vi "CheckState.vi"(8 "Error In":errorcluster, 10 "With sound?":bool, 11 "Droid in":refnum<class "Droid.lvclass">) -> (0 "Error Out":errorcluster, 3 "Droid out":refnum<class "Droid.lvclass">)   [LabVIEW 2021, in "Droid.lvclass"]
uses:
  Droid.lvclass
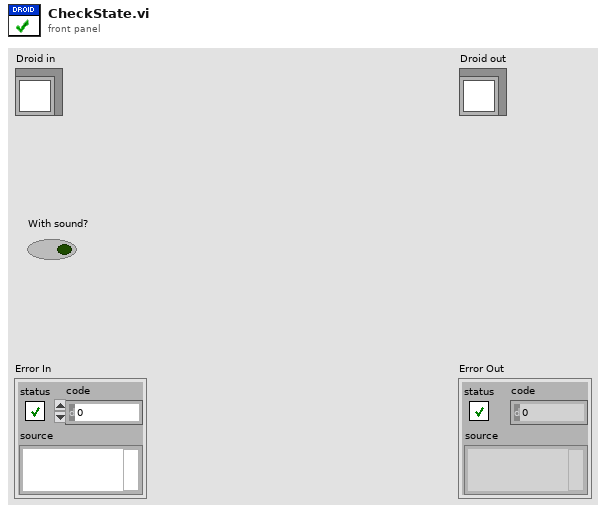
[diagram p1: front panel]
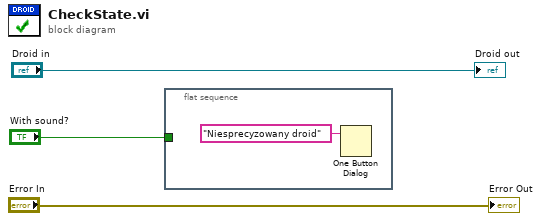
[diagram p0: block diagram]
diagram:
  n1 = flat-sequence {
    tunnel: "With sound?" -> [_]
    frame #0 {
      n2 = One Button Dialog(message="Niesprecyzowany droid") -> ()  [unwired: 1 in, 1 out]
    }
  }
  "Error Out" <- "Error In"
  "Droid out" <- "Droid in"
